vi "FlattenVariantToXMLBase64.vi"(8 "error in (no error)":errorcluster, 11 "Variant":variant) -> (0 "error out":errorcluster, 2 "data":u8[](array[numeric]), 3 "type string":u8[](array[numeric]))   [LabVIEW 2019, in "Custom Devices Storage.lvlib"]
uses:
  Custom Devices Storage.lvlib
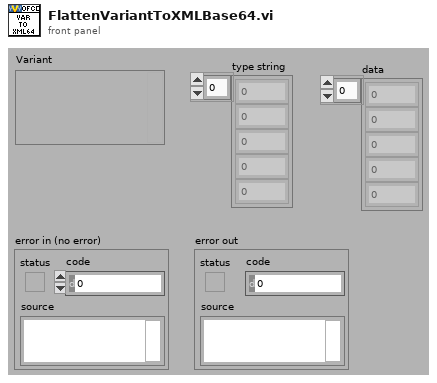
[diagram p1: front panel]
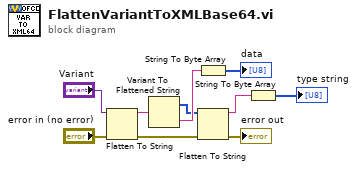
[diagram p0: block diagram]
diagram:
  n1 = Flatten To String(anything="Variant", error in (no error)="error in (no error)") -> (data string=w7:string, error out=w2:errorcluster)  [unwired: 2 in, 1 out]
  n2 = Variant To Flattened String(Variant=w7) -> (data string=w10:string, 1:w8:i16[])
  n3 = String To Byte Array(string=w10) -> (unsigned byte array=→"data":u8[])
  n4 = Flatten To String(anything=w8, error in (no error)=w2) -> (data string=w9:string, error out=→"error out":errorcluster)  [unwired: 2 in, 1 out]
  n5 = String To Byte Array(string=w9) -> (unsigned byte array=→"type string":u8[])
